vi "bgk_data_acquisition_loop_01_01.vi"(7 "Period (s)":dbl=600.0 caption="采样周期 (s)" format="%#_13g", 8 "error in (no error)":errorcluster caption="错误输入（无错误）", 11 "Message Queues":T1 caption="消息队列") -> (0 "error out":errorcluster caption="错误输出")   [LabVIEW 2015]
uses:
  message_queue/all_rt_message_queues.ctl
  message_queue/message_cluster.ctl
  <vilib>/Platform/TimedLoop/XDataNode/timing_clust.ctl
  <vilib>/Platform/TimedLoop/XDataNode/nitl_modes.ctl
  <vilib>/Platform/TimedLoop/XDataNode/wakeup.ctl
  <vilib>/Platform/TimedLoop/XDataNode/loadnilvce.vi
  <vilib>/Instr/_visa.llb/VISA Configure Serial Port (Instr).vi
  globals/global_all_rt_loop_stop.vi
  <vilib>/Platform/TimedLoop/XDataNode/XDataNode.xnode
  <vilib>/Platform/TimedLoop/XDataNode/XDNodeRunTimeDep.lvlib
  message_queue/message_queue.lvlib
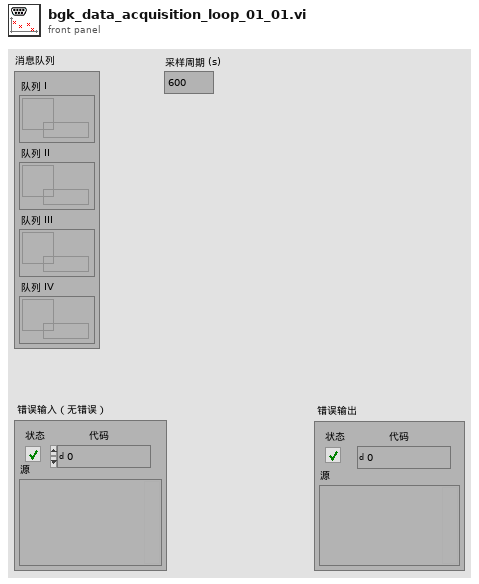
[diagram p1: front panel]
types:
  T1 = typedef "message_queue.lvlib/all_rt_message_queues.ctl" = cluster{"Queue I":refnum<queue>, "Queue II":refnum<queue>, "Queue III":refnum<queue>, "Queue IV":refnum<queue>}
  T2 = typedef "XDNodeRunTimeDep.lvlib/timing_clust.ctl" = cluster{"Expected End [f-1]":u64, "Actual End [f-1]":u64, "Finished Late? [f-1]":bool, "Expected End [i-1]":u64, "Actual End [i-1]":u64, "Finished Late? [i-1]":bool, "Expected Start [i]":u64, "Actual Start [i]":u64, "Expected Start [f]":u64, "Actual Start [f]":u64, "Source Name":string, "Structure Name":string, "Period":i64, "Deadline":i64, "Offset":i64, "Start":i64, "Priority":i32, "Timeout":i32, "Mode":T3, "Wakeup Reason":T4, "Error":errorcluster, "Source Type":string, "Secondary Source Type":string, "Global End Time":u64, "Global Start Time":u64, "Frame Duration":u64, "Iteration Duration":u64, "Assigned CPU":i32, "I/O Scan Engine Mode":u32}
  T3 = typedef "XDNodeRunTimeDep.lvlib/nitl_modes.ctl" = enum32{"No Change", "Process missed periods, maintain original phase", "Discard missed periods, maintain original phase", "Process missed periods, ignore original phase", "Discard missed periods, ignore original phase"}
  T4 = typedef "XDNodeRunTimeDep.lvlib/wakeup.ctl" = enum32{"Normal", "Aborted", "Asynchronous wakeup", "Timing source error", "Timed loop error", "Timeout"}
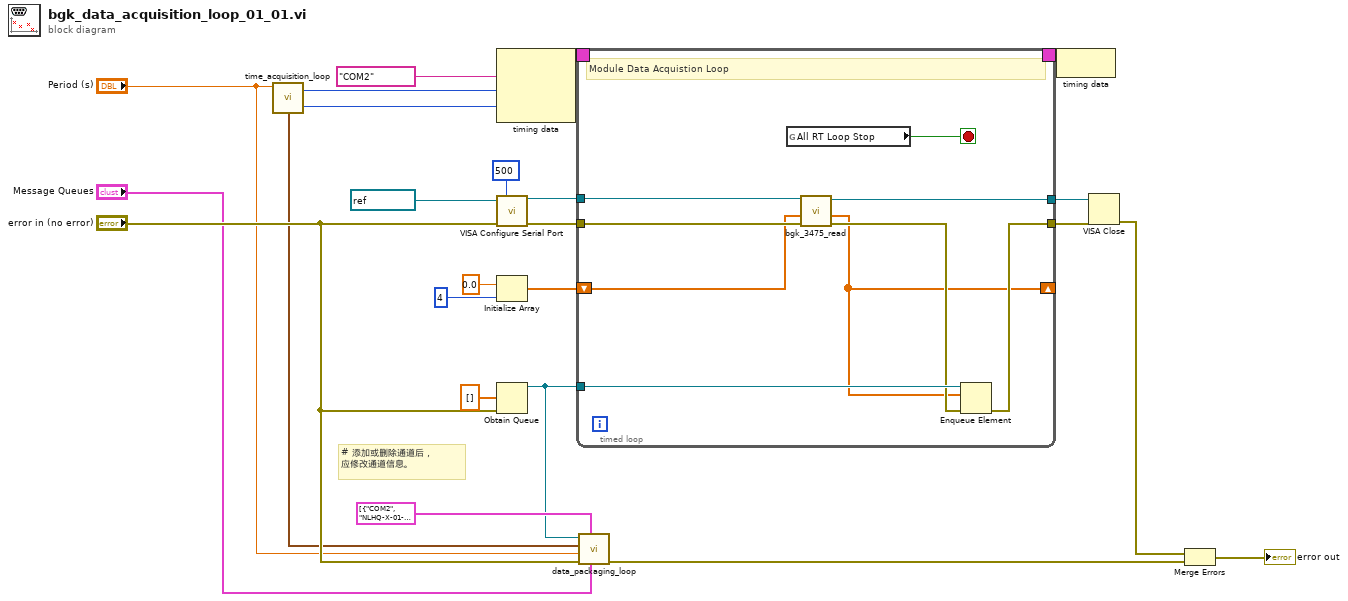
[diagram p0: block diagram]
diagram:
  # "# 添加或删除通道后，\n应修改通道信息。"
  n1 = call "time_acquisition_loop.vi"("Period (s)"="Period (s)") -> ("t0 (scan)"=w3:i64, "Period (scan)"=w4:i64, "timestamp output"=w2:timestamp)  [unwired: 4 in]
  n2 = node-c288("COM2" ("Structure Name"), w4, w3) -> (w23:T2)
  n3 = call-poly "VISA Configure Serial Port"("VISA resource name"=refnum<visa-resource-name> "COM2", "timeout (10sec)"=u32 500, "error in (no error)"="error in (no error)") -> ("VISA resource name out"=w16:refnum<visa-resource-name>, "error out"=w20:errorcluster)  [unwired: 11 in]
  n4 = Initialize Array(0.0 ("元素"), 4 ("维数大小")) -> (w6:dbl[])
  n5 = Obtain Queue(element data type=dbl[] [] ("数据类型"), error in (no error)="error in (no error)") -> (queue out=w9:refnum<queue>)  [unwired: 3 in, 2 out]
  n6 = timed-loop {
    timing: w23 -> [_]
    timing-out: [_] -> w22
    tunnel: w9 -> [w32]
    tunnel: w20 -> [w27]
    tunnel: [w31] -> w18
    tunnel: [w30] -> w19
    tunnel: w16 -> [w28]
    shift-right: [w25] -> _
    shift-left: w6 -> [w26]
    stop <- w33 stop-if-true
    # "Module Data Acquistion Loop"
    n7 = global read "global_all_rt_loop_stop.vi" "All RT Loop Stop"() -> (w33:bool)
    n8 = call "bgk_3475_read.vi"("error in (no error)"=w27, "Last Data Array"=w26, "VISA Ref Input"=w28) -> ("error out"=w29:errorcluster, "New Data Array"=w25:dbl[], "VISA Ref Output"=w30:refnum<visa-resource-name>)  [unwired: 6 in]
    n9 = Enqueue Element(queue=w32, element=w25, error in (no error)=w29) -> (error out=w31:errorcluster)  [unwired: 1 in, 2 out]
  }
  n10 = call "data_packaging_loop.vi"("Message Queues"="Message Queues", "channel info array"=cluster{"Module":string, "Channel":string}[] [{"Module"="COM2", "Channel"="NLHQ-X-01-D01"}, {"Module"="COM2", "Channel"="NLHQ-X-02-D01"}, {"Module"="COM2", "Channel"="NLHQ-X-04-D01"}, {"Module"="COM2", "Channel"="NLHQ-X-06-D01"}], "error in (no error)"="error in (no error)", "sampling period (s)"="Period (s)", "timestamp"=w2, "data queue"=w9) -> ("error out"=w12:errorcluster)  [unwired: 5 in]
  n11 = node-c288(w22) -> ()
  n12 = VISA Close(VISA resource name=w19, error in (no error)=w18) -> (error out=w17:errorcluster)
  n13 = Merge Errors(w17, w12) -> (→"error out":errorcluster)
